vi "support_locateReportFolder.vi"(8 "error in (no error)":errorcluster, 11 "pdbm_general_report_info":refnum<vi>) -> (0 "error IO":errorcluster, 3 "Report Folder path":path)   [LabVIEW 2011]
doc: "retrieves Report root folder.\n---------------------------------------------------------------\nAuthor: Dang Lam\nEmail: danglamtd@gmail.com"
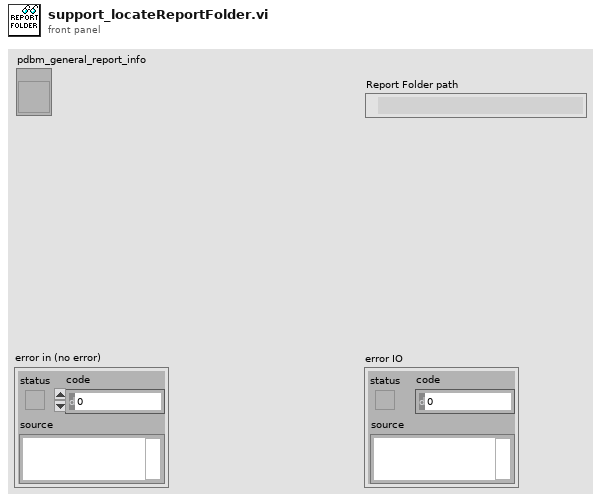
[diagram p1: front panel]
types:
  T1 = cluster{"Operator":string, "Customer":string, "Report":path, "UUT Serial Number":string, "Sale Order Number":string}
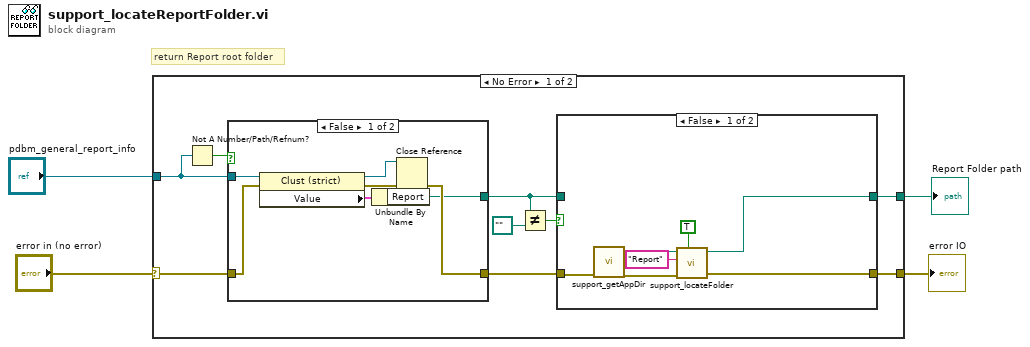
[diagram p0: block diagram]
diagram:
  # "return Report root folder"
  n1 = case shown="No Error" "error in (no error)" {
    selector: "error in (no error)" -> [w13 w31]
    tunnel: [w6 w31] -> w3
    tunnel: "pdbm_general_report_info" -> [w12 _]
    tunnel: [w5 _] -> w1
    frame No Error {
      n2 = Not A Number/Path/Refnum?(number/path/refnum=w12) -> (NaN/Path/Refnum?=w11:bool)
      n3 = case shown="False" w11 {
        tunnel: w13 -> [w29 w30]
        tunnel: w12 -> [w26 _]
        tunnel: [w24 w30] -> w7
        tunnel: [w23 _] -> w8
        frame False {
          n4 = property class="Clust (strict)"(reference=w26, error in=w29) -> (reference out=w27:refnum<vi>, error out=w28:errorcluster, "Value"=w25:T1)
          n5 = Unbundle By Name(w25) -> ("Report"=w23:path)
          n6 = Close Reference(reference=w27, error in (no error)=w28) -> (error out=w24:errorcluster)
        }
        frame True {
        }
      }
      n7 = Not Equal?(x=w8, y=path "") -> (x != y?=w9:bool)
      n8 = case shown="False" w9 {
        tunnel: w8 -> [_ w22]
        tunnel: [w15 w22] -> w5
        tunnel: w7 -> [w20 w21]
        tunnel: [w14 w21] -> w6
        frame False {
          n9 = call "support_getAppDir.vi"("error in (no error)"=w20) -> ("error out"=w19:errorcluster, "App.Dir"=w18:path)  [unwired: 9 in]
          n10 = call "support_locateFolder.vi"("create if not found?"=TRUE, "error in (no error)"=w19, "Folder"="Report" ("folder"), "Root"=w18) -> ("error IO"=w14:errorcluster, "path"=w15:path)  [unwired: 5 in, 1 out]
        }
        frame True {
        }
      }
    }
    frame Error {
    }
  }
  "error IO" <- w3
  "Report Folder path" <- w1
